vi "1Decembre2016.vi"() -> ()   [LabVIEW 2014]
panel:
  out "XY Graph":T1(graph)
  out "Distance en Block":i32
  out "Distance O-E":i32
  out "Direction":u16(ring) items=["Ouest", "Est", "Sud", "Nord"]
  out "Distance N-S":i32
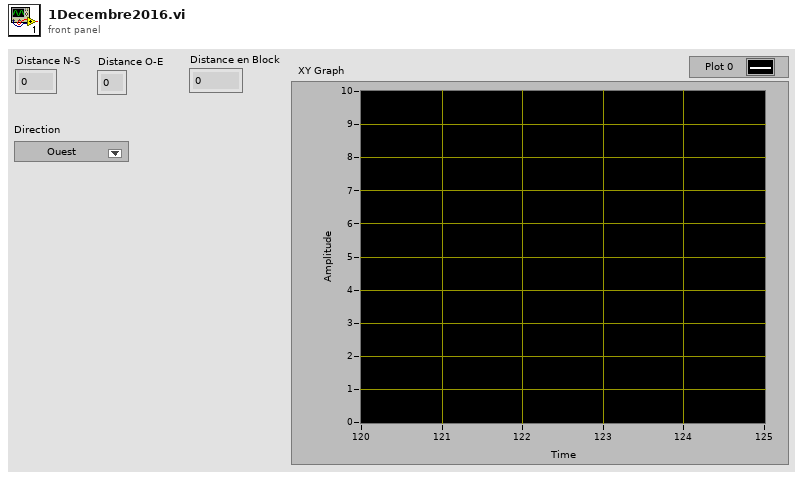
[diagram p1: front panel]
types:
  T1 = cluster{"Distance O-E":i32, "Distance N-S":i32}[]
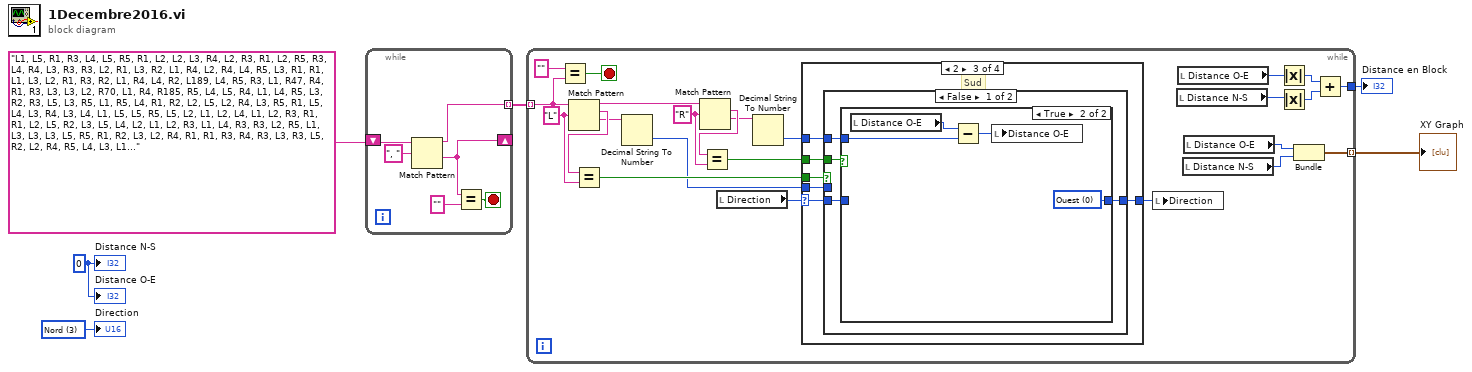
[diagram p0: block diagram]
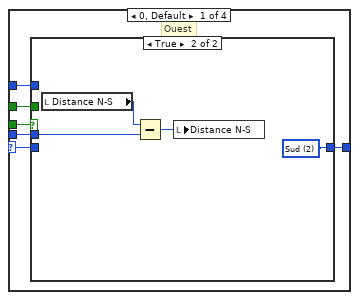
[diagram p2: hidden frame]
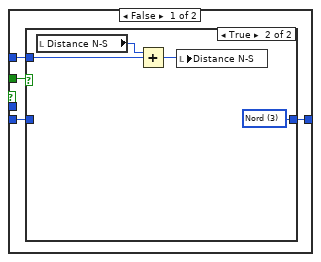
[diagram p3: hidden frame]
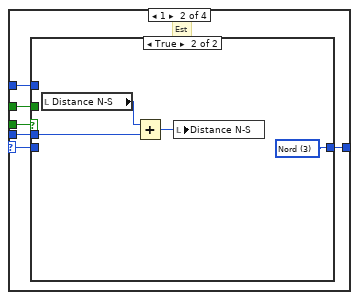
[diagram p5: hidden frame]
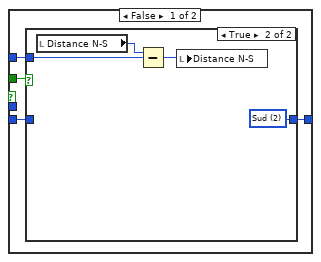
[diagram p6: hidden frame]
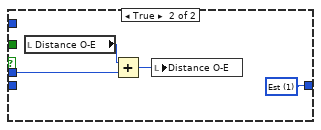
[diagram p9: hidden frame]
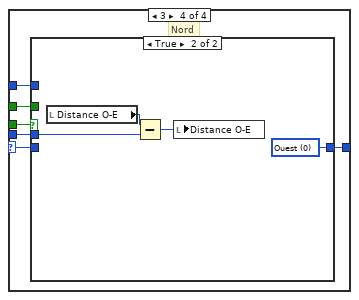
[diagram p10: hidden frame]
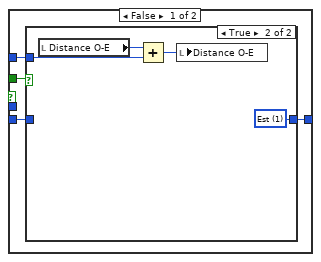
[diagram p11: hidden frame]
diagram:
  w4 = 0 ("Distance N-S")
  w3 = u16 3 items=["Ouest", "Est", "Sud", "Nord"] ("Direction Actuel")
  n1 = while {
    shift-right: [w8] -> _
    shift-left: "L1, L5, R1, R3, L4, L5, R5, R1, L2, L2, L3, R4, L2, R3, R1, L2, R5, R3, L4, R4, L3, R3, R3, L2, R1, L3, R2, L1, R4, L2, R4, L4, R5, L3, R1, R1, L1, L3, L2, R1, R3, R2, L1, R4, L4, R2, L189, L4, R5, R3, L1, R47, R4, R1, R3, L3, L3, L2, R70, L1, R4, R185, R5, L4, L5, R4, L1, L4, R5, L3, R2, R3, L5, L3, R5, L1, R5, L4, R1, R2, L2, L5, L2, R4, L3, R5, R1, L5, L4, L3, R4, L3, L4, L1, L5, L5, R5, L5, L2, L1, L2, L4, L1, L2, R3, R1, R1, L2, L5, R2, L3, L5, L4, L2, L1, L2, R3, L1, L4, R3, R3, L2, R5, L1, L3, L3, L3, L5, R5, R1, R2, L3, L2, R4, R1, R1, R3, R4, R3, L3, R3, L5, R2, L2, R4, R5, L4, L3, L1, L5, L1, R1, R2, L1, R3, R4, R5, R2, R3, L2, L1, L5" -> [w12]
    tunnel: [w10] -> w5 mode=indexing
    stop <- w9 stop-if-true
    n2 = Match Pattern(string=w12, regular expression=", ") -> (before substring=w10:string, after substring=w8:string)  [unwired: 1 in, 2 out]
    n3 = Equal?(x=w8, y="") -> (x = y?=w9:bool)
  }
  n4 = while {
    tunnel: w5 -> [w29] mode=indexing
    tunnel: [w16] -> w2
    tunnel: [w13] -> w1 mode=indexing
    stop <- w30 stop-if-true
    w33 = "R"
    w34 = "L"
    n5 = Equal?(x="" ("y"), y=w29) -> (x = y?=w30:bool)
    n6 = Match Pattern(string=w29, regular expression=w34) -> (before substring=w36:string, match substring=w35:string, after substring=w24:string)  [unwired: 1 in, 1 out]
    n7 = Equal?(x=w35, y=w34) -> (x = y?=w27:bool)
    n8 = Decimal String To Number(string=w24) -> (number=w23:i32)  [unwired: 2 in, 1 out]
    n9 = Match Pattern(string=w36, regular expression=w33) -> (match substring=w32:string, after substring=w25:string)  [unwired: 1 in, 2 out]
    n10 = Equal?(x=w32, y=w33) -> (x = y?=w26:bool)
    n11 = local read "Direction"() -> (w28:u16)
    n12 = Decimal String To Number(string=w25) -> (number=w22:i32)  [unwired: 2 in, 1 out]
    n13 = case shown="2" w28 {
      selector: w28 -> [w40 w59 w78 w97]
      tunnel: w27 -> [w42 w61 w80 w99]
      tunnel: w26 -> [w37 w56 w75 w94]
      tunnel: [w41 w60 w79 w98] -> w21
      tunnel: w23 -> [w39 w58 w77 w96]
      tunnel: w22 -> [w38 w57 w76 w95]
      frame 0, Default {
        # "Ouest"
        n14 = case shown="True" w42 {
          tunnel: [w44 w54] -> w41
          tunnel: w40 -> [w45 _]
          tunnel: w39 -> [_ w52]
          tunnel: w38 -> [w43 _]
          tunnel: w37 -> [w46 _]
          frame False {
            n15 = case shown="True" w46 {
              tunnel: w45 -> [w47 _]
              tunnel: [w47 w51] -> w44
              tunnel: w43 -> [_ w48]
              frame False {
              }
              frame True {
                w51 = u16 3 items=["Ouest", "Est", "Sud", "Nord"] ("Direction Actuel")
                n16 = local read "Distance N-S"() -> (w49:i32)
                n17 = Add(x=w49, y=w48) -> (x+y=w50:i32)
                n18 = local write "Distance N-S"(w50) -> ()
              }
            }
          }
          frame True {
            w54 = u16 2 items=["Ouest", "Est", "Sud", "Nord"] ("Direction Actuel")
            n19 = local read "Distance N-S"() -> (w53:i32)
            n20 = Subtract(x=w53, y=w52) -> (x-y=w55:i32)
            n21 = local write "Distance N-S"(w55) -> ()
          }
        }
      }
      frame 1 {
        # "Est"
        n22 = case shown="True" w61 {
          tunnel: [w63 w73] -> w60
          tunnel: w59 -> [w64 _]
          tunnel: w58 -> [_ w71]
          tunnel: w57 -> [w62 _]
          tunnel: w56 -> [w65 _]
          frame False {
            n23 = case shown="True" w65 {
              tunnel: w64 -> [w66 _]
              tunnel: [w66 w70] -> w63
              tunnel: w62 -> [_ w67]
              frame False {
              }
              frame True {
                w70 = u16 2 items=["Ouest", "Est", "Sud", "Nord"] ("Direction Actuel")
                n24 = local read "Distance N-S"() -> (w68:i32)
                n25 = Subtract(x=w68, y=w67) -> (x-y=w69:i32)
                n26 = local write "Distance N-S"(w69) -> ()
              }
            }
          }
          frame True {
            w73 = u16 3 items=["Ouest", "Est", "Sud", "Nord"] ("Direction Actuel")
            n27 = local read "Distance N-S"() -> (w72:i32)
            n28 = Add(x=w72, y=w71) -> (x+y=w74:i32)
            n29 = local write "Distance N-S"(w74) -> ()
          }
        }
      }
      frame 2 {
        # "Sud"
        n30 = case shown="False" w80 {
          tunnel: [w82 w92] -> w79
          tunnel: w78 -> [w83 _]
          tunnel: w77 -> [_ w90]
          tunnel: w76 -> [w81 _]
          tunnel: w75 -> [w84 _]
          frame False {
            n31 = case shown="True" w84 {
              tunnel: w83 -> [w85 _]
              tunnel: [w85 w89] -> w82
              tunnel: w81 -> [_ w86]
              frame False {
              }
              frame True {
                w89 = u16 0 items=["Ouest", "Est", "Sud", "Nord"] ("Direction Actuel")
                n32 = local read "Distance O-E"() -> (w87:i32)
                n33 = Subtract(x=w87, y=w86) -> (x-y=w88:i32)
                n34 = local write "Distance O-E"(w88) -> ()
              }
            }
          }
          frame True {
            w92 = u16 1 items=["Ouest", "Est", "Sud", "Nord"] ("Direction Actuel")
            n35 = local read "Distance O-E"() -> (w91:i32)
            n36 = Add(x=w91, y=w90) -> (x+y=w93:i32)
            n37 = local write "Distance O-E"(w93) -> ()
          }
        }
      }
      frame 3 {
        # "Nord"
        n38 = case shown="True" w99 {
          tunnel: [w101 w111] -> w98
          tunnel: w97 -> [w102 _]
          tunnel: w96 -> [_ w109]
          tunnel: w95 -> [w100 _]
          tunnel: w94 -> [w103 _]
          frame False {
            n39 = case shown="True" w103 {
              tunnel: w102 -> [w104 _]
              tunnel: [w104 w108] -> w101
              tunnel: w100 -> [_ w106]
              frame False {
              }
              frame True {
                w108 = u16 1 items=["Ouest", "Est", "Sud", "Nord"] ("Direction Actuel")
                n40 = local read "Distance O-E"() -> (w105:i32)
                n41 = Add(x=w105, y=w106) -> (x+y=w107:i32)
                n42 = local write "Distance O-E"(w107) -> ()
              }
            }
          }
          frame True {
            w111 = u16 0 items=["Ouest", "Est", "Sud", "Nord"] ("Direction Actuel")
            n43 = local read "Distance O-E"() -> (w110:i32)
            n44 = Subtract(x=w110, y=w109) -> (x-y=w112:i32)
            n45 = local write "Distance O-E"(w112) -> ()
          }
        }
      }
    }
    n46 = local write "Direction"(w21) -> ()
    n47 = local read "Distance N-S"() -> (w18:i32)
    n48 = local read "Distance O-E"() -> (w20:i32)
    n49 = local read "Distance N-S"() -> (w14:i32)
    n50 = local read "Distance O-E"() -> (w15:i32)
    n51 = Absolute Value(x=w20) -> (abs(x)=w19:i32)
    n52 = Absolute Value(x=w18) -> (abs(x)=w17:i32)
    n53 = Bundle("Distance O-E"=w15, "Distance N-S"=w14) -> (w13:cluster{"Distance O-E":i32, "Distance N-S":i32})  [unwired: 1 in]
    n54 = Add(x=w19, y=w17) -> (x+y=w16:i32)
  }
  "Distance en Block" <- w2
  "XY Graph" <- w1
  "Distance N-S" <- w4
  "Direction" <- w3
  "Distance O-E" <- w4
